vi "Add Calculate Channel_Minimum_Minimum.vi"(7 "SysDef Ref":T1, 8 "error in (error out)":errorcluster, 9 "Minimum Settings":T2, 11 "Calculated Channels Ref":refnum<k24>) -> (0 "error out":errorcluster, 3 "Calculated Channels Ref Out":refnum<k24>)   [LabVIEW 2019, in "Simple SysDef API.lvlib"]
uses:
  <userlib>/SimpleSysDef/Simple SysDef API.lvlib
  NationalInstruments.VeriStand.SystemDefinitionAPI
  <userlib>/SimpleSysDef/_SubVIs/Add Calculate Channel_Maximum_Settings.ctl
  <userlib>/SimpleSysDef/_SubVIs/System Definition Reference.ctl
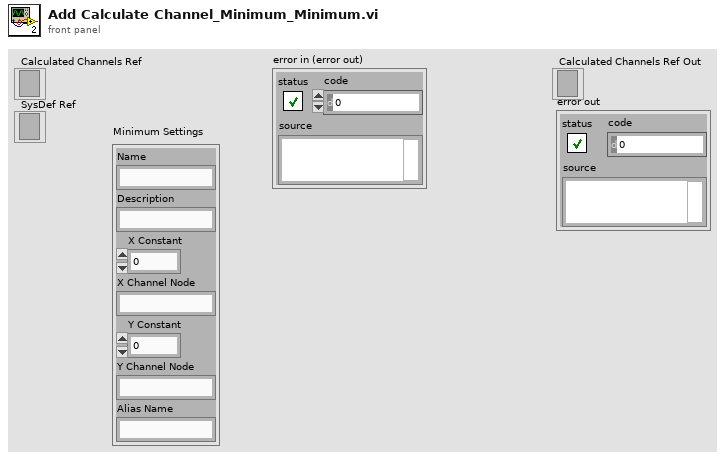
[diagram p1: front panel]
types:
  T1 = typedef "Simple SysDef API.lvlib/System Definition Reference.ctl" = refnum<k24>
  T2 = typedef "Simple SysDef API.lvlib/Add Calculate Channel_Maximum_Settings.ctl" = cluster{"Name":string, "Description":string, "X Constant":dbl, "X Channel Node":string, "Y Constant":dbl, "Y Channel Node":string, "Alias Name":string}
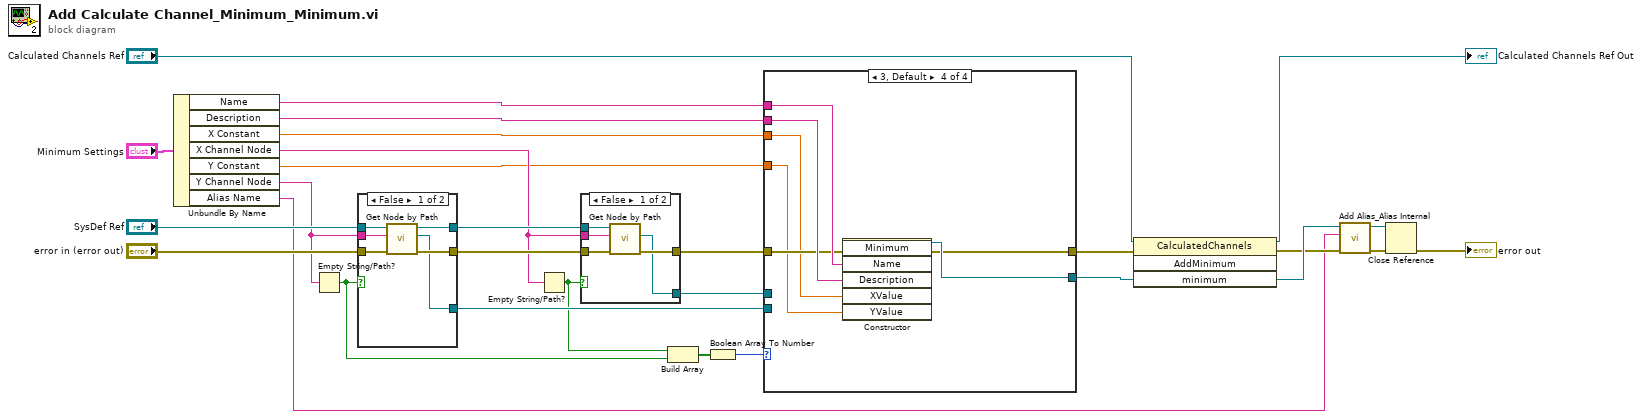
[diagram p0: block diagram]
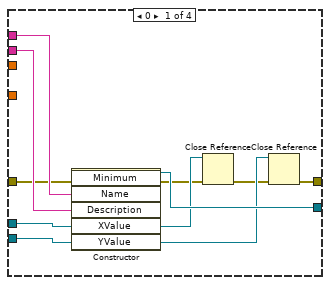
[diagram p2: hidden frame]
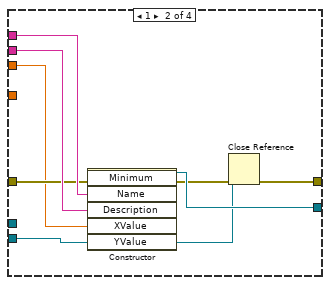
[diagram p3: hidden frame]
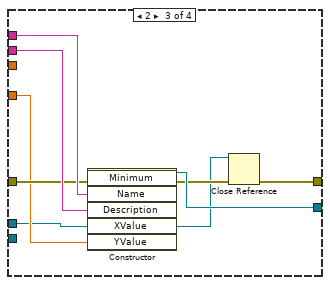
[diagram p4: hidden frame]
diagram:
  n1 = Unbundle By Name("Minimum Settings") -> ("Name"=w23:string, "Description"=w22:string, "X Constant"=w7:dbl, "X Channel Node"=w13:string, "Y Constant"=w6:dbl, "Y Channel Node"=w18:string, "Alias Name"=w1:string)
  n2 = Empty String/Path?(string/path=w18) -> (empty?=w11:bool)
  n3 = case shown="False" w11 {
    tunnel: "error in (error out)" -> [w33 w35]
    tunnel: [w32 w35] -> w16
    tunnel: "SysDef Ref" -> [w31 w34]
    tunnel: [w30 w34] -> w17
    tunnel: [w29 _] -> w19
    tunnel: w18 -> [w28 _]
    frame False {
      n4 = call <userlib>:"Get Node by Path.vi"("error in (no error)"=w33, "System Definition Node Path"=w28, "SysDef Ref"=w31) -> ("error out"=w32:errorcluster, "Node Ref"=w29:refnum<k24>, "SysDef Ref Out"=w30:T1)  [unwired: 6 in]
    }
    frame True {
    }
  }
  n5 = Empty String/Path?(string/path=w13) -> (empty?=w12:bool)
  n6 = case shown="False" w12 {
    tunnel: w16 -> [w40 w41]
    tunnel: [w39 w41] -> w14
    tunnel: w17 -> [w38 _]
    tunnel: [w37 _] -> w15
    tunnel: w13 -> [w36 _]
    frame False {
      n7 = call <userlib>:"Get Node by Path.vi"("error in (no error)"=w40, "System Definition Node Path"=w36, "SysDef Ref"=w38) -> ("error out"=w39:errorcluster, "Node Ref"=w37:refnum<k24>)  [unwired: 6 in, 1 out]
    }
    frame True {
    }
  }
  n8 = Build Array(w12, w11) -> (w10:bool[])
  n9 = Boolean Array To Number(Boolean array=w10) -> (number=w9:u32)
  n10 = case shown="3, Default" w9 {
    tunnel: [w42 w53 w62 w68] -> w8
    tunnel: [w50 w58 w66 w73] -> w5
    tunnel: w23 -> [w49 w57 w65 w72]
    tunnel: w22 -> [w48 w56 w64 w71]
    tunnel: w19 -> [w45 w54 _ _]
    tunnel: w15 -> [w46 _ w59 _]
    tunnel: w14 -> [w47 w55 w63 w70]
    tunnel: w7 -> [_ w51 _ w69]
    tunnel: w6 -> [_ _ w60 w67]
    frame 0 {
      n11 = constructor class="Minimum"(error in=w47, "Name"=w49, "Description"=w48, "XValue"=w46, "YValue"=w45) -> (reference out=w50:refnum<k24>, error out=w43:errorcluster)  [unwired: 2 in, 5 out]
      n12 = Close Reference(reference=w46, error in (no error)=w43) -> (error out=w44:errorcluster)
      n13 = Close Reference(reference=w45, error in (no error)=w44) -> (error out=w42:errorcluster)
    }
    frame 1 {
      n14 = constructor class="Minimum"(error in=w55, "Name"=w57, "Description"=w56, "XValue"=w51, "YValue"=w54) -> (reference out=w58:refnum<k24>, error out=w52:errorcluster)  [unwired: 2 in, 5 out]
      n15 = Close Reference(reference=w54, error in (no error)=w52) -> (error out=w53:errorcluster)
    }
    frame 2 {
      n16 = constructor class="Minimum"(error in=w63, "Name"=w65, "Description"=w64, "XValue"=w59, "YValue"=w60) -> (reference out=w66:refnum<k24>, error out=w61:errorcluster)  [unwired: 2 in, 5 out]
      n17 = Close Reference(reference=w59, error in (no error)=w61) -> (error out=w62:errorcluster)
    }
    frame 3, Default {
      n18 = constructor class="Minimum"(error in=w70, "Name"=w72, "Description"=w71, "XValue"=w69, "YValue"=w67) -> (reference out=w73:refnum<k24>, error out=w68:errorcluster)  [unwired: 2 in, 5 out]
    }
  }
  n19 = invoke class="CalculatedChannels" method="AddMinimum"(reference="Calculated Channels Ref", error in=w8, "minimum"=w5) -> (reference out=→"Calculated Channels Ref Out":refnum<k24>, error out=w4:errorcluster)  [unwired: 1 in, 2 out]
  n20 = call <userlib>:"Add Alias_Alias Internal.vi"("error in (no error)"=w4, "Name"=w1, "Base Node"=w5) -> ("error out"=w3:errorcluster, "Base Node out"=w2:refnum<k24>)  [unwired: 7 in]
  n21 = Close Reference(reference=w2, error in (no error)=w3) -> (error out=→"error out":errorcluster)
